vi "Change flat sequnce size.vi"   [LabVIEW 2015]
uses:
  <vilib>/Utility/miscctls.llb/LVBoundsTypeDef.ctl
types:
  T1 = typedef "LVBoundsTypeDef.ctl" = cluster{"Width":u32, "Height":u32}
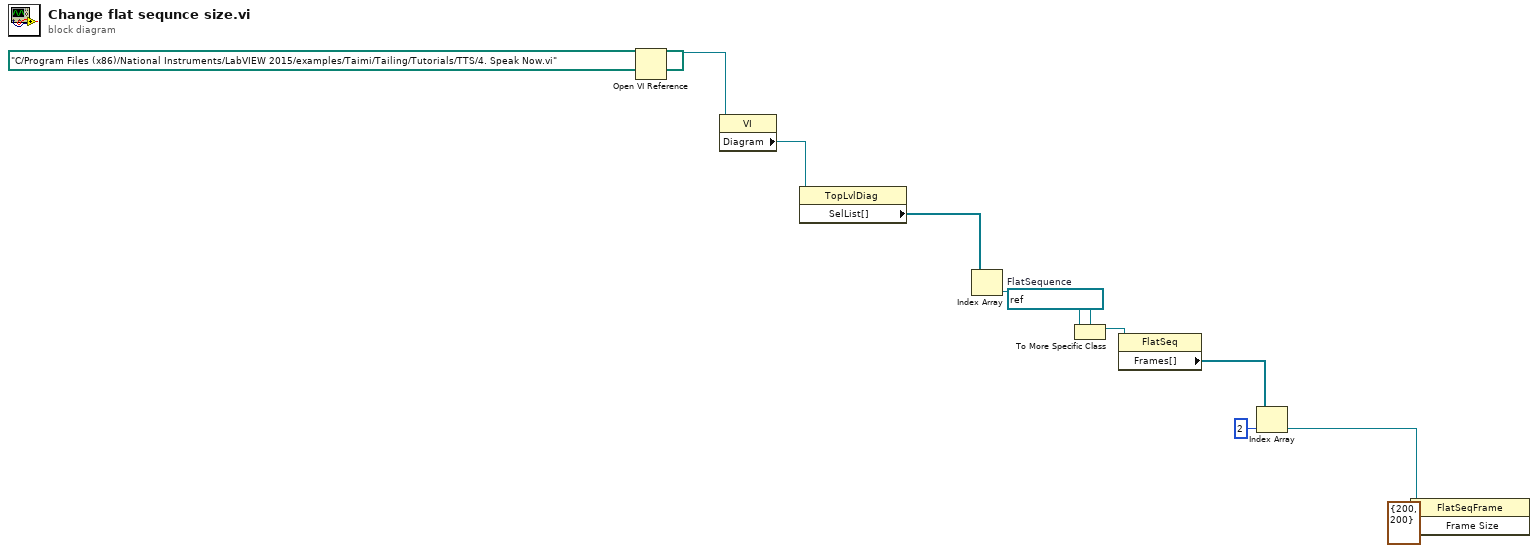
[diagram p0: block diagram]
diagram:
  w6 = refnum<vi> refnum  # FlatSequence
  n1 = Open VI Reference(vi path=path "C:/Program Files (x86)/National Instruments/LabVIEW 2015/examples/Taimi/Tailing/Tutorials/TTS/4. Speak Now.vi") -> (vi reference=w10:refnum<vi>)  [unwired: 5 in, 1 out]
  n2 = property class="VI"(reference=w10) -> ("Diagram"=w9:refnum<vi>)  [unwired: 1 in, 2 out]
  n3 = property class="TopLvlDiag"(reference=w9) -> ("SelList[]"=w8:refnum<vi>[])  [unwired: 1 in, 2 out]
  n4 = Index Array(array=w8) -> (element=w7:refnum<vi>)  [unwired: 1 in]
  n5 = To More Specific Class(target class=w6, reference=w7) -> (specific class reference=w5:refnum<vi>)  [unwired: 1 in, 1 out]
  n6 = property class="FlatSeq"(reference=w5) -> ("Frames[]"=w4:refnum<vi>[])  [unwired: 1 in, 2 out]
  n7 = Index Array(array=w4, index=2) -> (element=w2:refnum<vi>)
  n8 = property class="FlatSeqFrame"(reference=w2, "Frame Size"=T1 {"Width"=200, "Height"=200}) -> ()  [unwired: 1 in, 2 out]
